vi "TEST - Set VI Top Level.vi"(8 "error in (no error)":errorcluster) -> (0 "error out":errorcluster, 2 "pass":bool)   [LabVIEW 2020]
uses:
  <userlib>/_OpenG.lib/error/error.llb/openg_error.lvlib
  source/library/openg_file.lvlib
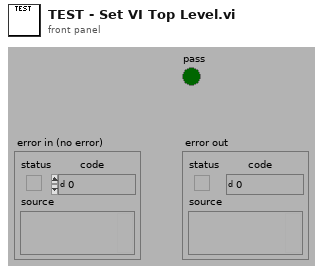
[diagram p1: front panel]
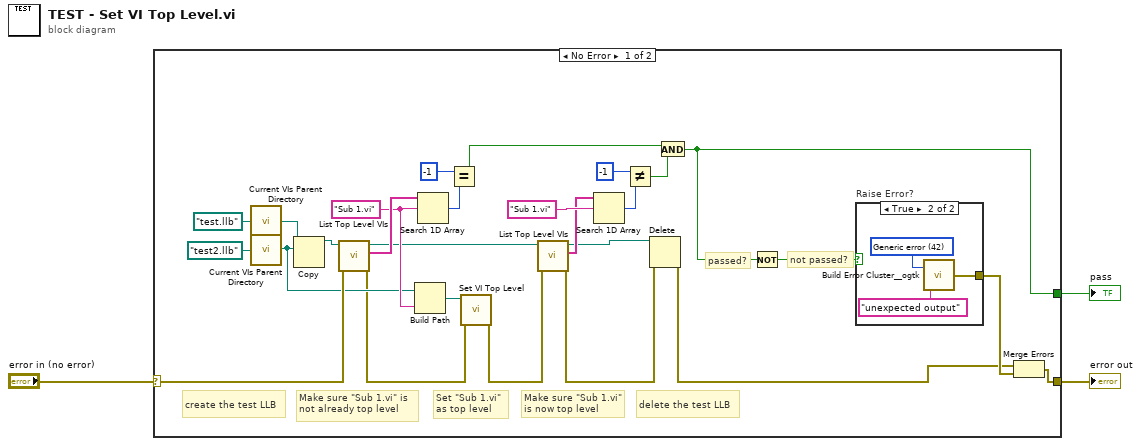
[diagram p0: block diagram]
diagram:
  n1 = case shown="No Error" "error in (no error)" {
    selector: "error in (no error)" -> [w26 w34]
    tunnel: [w7 _] -> w3
    tunnel: [w30 w34] -> w1
    frame No Error {
      w19 = "Sub 1.vi" ("String")
      # "create the test LLB"
      # "delete the test LLB"
      # "Make sure \"Sub 1.vi\" is now top level"
      # "Make sure \"Sub 1.vi\" is not already top level"
      # "Set \"Sub 1.vi\" as top level"
      # "not passed?"
      # "passed?"
      n2 = call "Current VIs Parent Directory.vi"("Relative path (.)"=path "test.llb") -> ("Parent Directory (+ Relative)"=w25:path)  [unwired: 4 in]
      n3 = call "Current VIs Parent Directory.vi"("Relative path (.)"=path "test2.llb") -> ("Parent Directory (+ Relative)"=w18:path)  [unwired: 4 in]
      n4 = Copy(10:w18, 11:w25) -> (3:w23:path)  [unwired: 3 in, 2 out]
      n5 = call "List Top Level VIs.vi"("error in (no error)"=w26, "LLB Path"=w23) -> ("error out"=w17:errorcluster, "Top-Level VIs"=w22:string[], "dup LLB Path"=w11:path)  [unwired: 7 in]
      n6 = Build Path(base path=w18, name or relative path=w19) -> (appended path=w16:path)
      n7 = Search 1D Array(1D array=w22, element=w19) -> (index of element=w21:i32)  [unwired: 1 in]
      n8 = Equal?(x=-1, y=w21) -> (x = y?=w8:bool)
      n9 = call "Set VI Top Level.vi"("error in (no error)"=w17, "VI Path"=w16) -> ("error out"=w10:errorcluster)  [unwired: 8 in, 1 out]
      n10 = call "List Top Level VIs.vi"("error in (no error)"=w10, "LLB Path"=w11) -> ("error out"=w5:errorcluster, "Top-Level VIs"=w12:string[], "dup LLB Path"=w6:path)  [unwired: 7 in]
      n11 = Search 1D Array(1D array=w12, element="Sub 1.vi" ("String")) -> (index of element=w13:i32)  [unwired: 1 in]
      n12 = Not Equal?(x=-1, y=w13) -> (x != y?=w9:bool)
      n13 = Delete(path (use dialog)=w6, error in=w5) -> (error out=w4:errorcluster)  [unwired: 3 in, 2 out]
      n14 = And(x=w8, y=w9) -> (x .and. y?=w7:bool)
      n15 = Not(x=w7) -> (.not. x?=w28:bool)
      n16 = case "Raise Error?" shown="True" w28 {
        tunnel: [_ w31] -> w29
        frame False {
        }
        frame True {
          w32 = 42 items=["No error", "Argument error", "Memory is full", "Out of zone", "End of file", "File already open", "Generic file I/O error", "File not found", "File permission error", "Disk is full", "Duplicate path", "Too many files open", "System feature not enabled", "Resource file not found", "Cannot add resource", "Resource not found", "Image not found", "Image memory error", "Pen does not exist", "Config type invalid", "Config token not found", "Config parse error", "Config memory error", "Bad external code format", "Bad external code offset", "External code not present", "Null window", "Destroy window error", "Null menu", "Print aborted", "Bad print record", "Print driver error", "Windows error during printing", "Memory error during printing", "Print dialog error", "Generic print error", "Invalid device refnum", "Device not found", "Device parameter error", "Device unit error", "Cannot open device", "Device call aborted", "Generic error", "Cancelled by user", "Object ID too low", "Object ID too high", "Object not in heap", "Unknown heap", "Unknown object (invalid DefProc)", "Unknown object (DefProc not in table)", "Message out of range", "Invalid (null) method", "Unknown message", "Manager call not supported", "Bad address", "Network operation in progress", "Network operation timed out", "Connection is busy", "Network attribute not supported", "Network error", "Address in use", "System out of memory", "Connection aborted", "Connection refused", "Not connected", "Already connected", "Connection closed", "Initialization error (interapplication manager)", "Bad occurrence", "Wait on unbound occurrence handler", "Occurrence queue overflow", "Datalog type conflict", "Unused", "Unrecognized type (interapplication manager)", "Memory corrupt", "Failed to make temporary DLL", "Old CIN version", "Drag socket not found", "Failed to load drop-object", "Failed to register OLE object", "Failed to release OLE object", "Format specifier type mismatch", "Unknown format specifier", "Too few format specifiers", "Too many format specifiers", "Scan failed", "Newer CIN version", "Error converting to variant", "Runtime menu error", "Password tampered", "Variant attribute not found", "Incompatible variant data type", "Event data is not available", "Event Store is not present", "Occurrence is not found", "Event Queue is not created", "Event info is not available", "Refnum passed is NULL", "Error retrieving Class GUID", "Error retrieving CoClass GUID", "Error retrieving TypeLib GUID.", "Bad built application magic bytes.", "Specific driver is different from the specific driver associated with the Logical Name.", "There is no session opened to the class driver.", "Max Error", "MAX - Error with config objects", "MAX - Error loading configuration", "MAX - Group not supported"]
          n17 = call <userlib>:"Build Error Cluster__ogtk.vi"("String to Prepend to source (\"\")"="unexpected output" ("String to Prepend to source (\"\")"), "code"=w32) -> ("error out"=w31:errorcluster)
        }
      }
      n18 = Merge Errors(w4, w29) -> (w30:errorcluster)
    }
    frame Error {
    }
  }
  "pass" <- w3
  "error out" <- w1
